vi "Read Configuration Class.vi"(8 "error in (no error)":errorcluster, 11 "Instrument in":refnum<class "Instrument.lvclass">) -> (0 "error out":errorcluster, 2 "Configuration.lvclass":refnum<class "Configuration.lvclass">, 3 "Instrument out":refnum<class "Instrument.lvclass">)   [LabVIEW 2016, in "Instrument.lvclass"]
uses:
  Instrument.lvclass
  Configuration/Configuration.lvclass
  Instrument.lvclass/Instrument.ctl
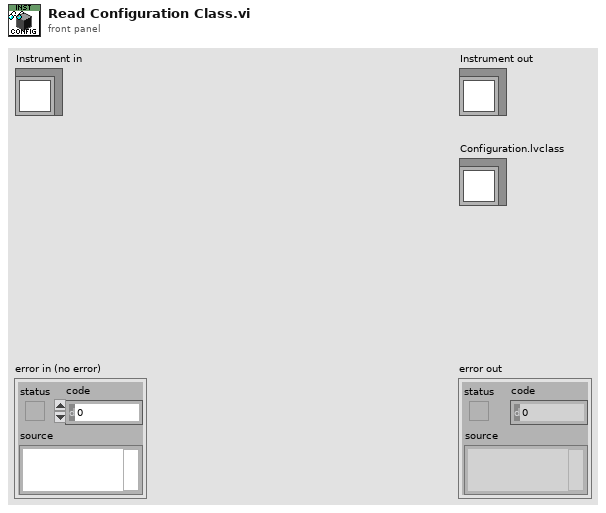
[diagram p1: front panel]
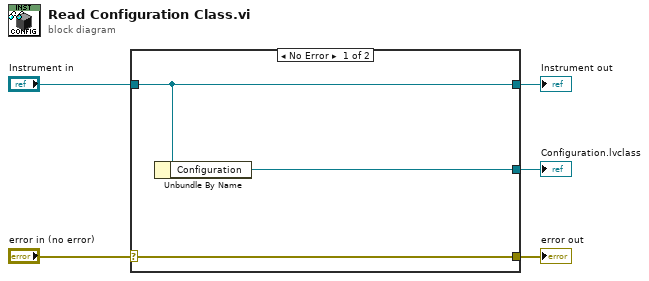
[diagram p0: block diagram]
diagram:
  n1 = case shown="No Error" "error in (no error)" {
    selector: "error in (no error)" -> [w8 w9]
    tunnel: [w8 w9] -> w4
    tunnel: [w7 w10] -> w2
    tunnel: "Instrument in" -> [w7 w10]
    tunnel: [w6 _] -> w1
    frame No Error {
      n2 = Unbundle By Name(w7) -> ("Configuration"=w6:refnum<class "Configuration.lvclass">)
    }
    frame Error {
    }
  }
  "error out" <- w4
  "Instrument out" <- w2
  "Configuration.lvclass" <- w1
